vi "Untitled 4.vi"() -> ()   [LabVIEW 2025]
panel:
  in  "IF Offset (V)":dbl=213.0
  in  "GPIB Addr (28)":refnum<visa-resource-name>="GPIB0::28::INSTR"
  in  "Center Freq (MHz)":dbl=213.0
  in  "Freq Span (kHz)":dbl=2000.0
  in  "RF Level (dBm)":dbl format="%#_13g"
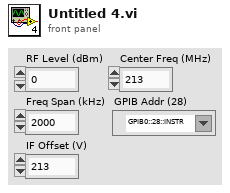
[diagram p1: front panel]
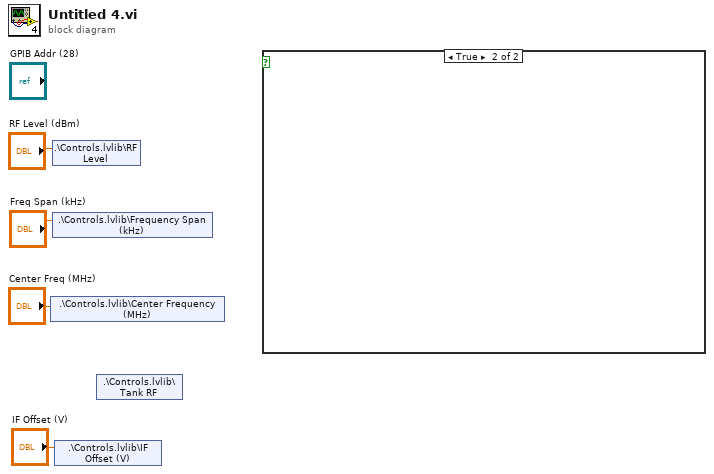
[diagram p0: block diagram]
diagram:
  n1 = shared-variable ".\\Controls.lvlib\\Center Frequency (MHz)"("Center Freq (MHz)") -> ()  [unwired: 1 in, 1 out]
  n2 = shared-variable ".\\Controls.lvlib\\RF Level"("RF Level (dBm)") -> ()  [unwired: 1 in, 1 out]
  n3 = shared-variable ".\\Controls.lvlib\\Frequency Span (kHz)"("Freq Span (kHz)") -> ()  [unwired: 1 in, 1 out]
  n4 = shared-variable ".\\Controls.lvlib\\IF Offset (V)"("IF Offset (V)") -> ()  [unwired: 1 in, 1 out]
  n5 = shared-variable ".\\Controls.lvlib\\Tank RF"() -> ()  [unwired: 1 in, 2 out]
  n6 = case shown="True" {
    selector: _ -> [_ _]
    frame False {
    }
    frame True {
    }
  }
